vi "vis_variables.vi"() -> ()   [LabVIEW 2017]
panel:
  out "Vis_Variables":T1
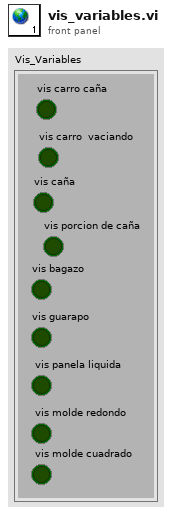
[diagram p1: front panel]
types:
  T1 = cluster{"vis carro caña":bool, "vis carro  vaciando":bool, "vis caña":bool, "vis porcion de caña":bool, "vis bagazo":bool, "vis guarapo":bool, " vis panela liquida":bool, " vis molde redondo":bool, " vis molde cuadrado":bool}
diagram:
